vi "combined arm safety.vi"(7 "Input":dbl) -> (8 "Safe Output":dbl, 13 "Safety Data":T1)   [LabVIEW 2013]
uses:
  typedefs/dashboard safety status data.ctl
  typedefs/fg_typedef.ctl
  typedefs/DevRef Type.ctl
  typedefs/subStates.ctl
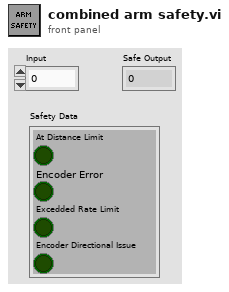
[diagram p1: front panel]
types:
  T1 = typedef "dashboard safety status data.ctl" = cluster{"At Distance Limit":bool, "Encoder Error":bool, "Excedded Rate Limit":bool, "Encoder Directional Issue":bool}
  T2 = typedef "subStates.ctl" = enum16{"null", "wait", "driver control", "auto", "manual override", "hold position", "rotate", "pickup", "pass", "load", "goto shoot", "shoot high goal", "shoot low goal", "cancel arm", "cancel shooter", "end", "test"}
  T3 = typedef "DevRef Type.ctl" = enum16{"Shooter Solenoid", "Latch Solenoid", "Right Up Sensor", "Right Down Sensor", "Hold Sensor", "2 Ball Switch", "Arm Encoder"}
  T4 = typedef "fg_typedef.ctl" = enum16{"Get", "Set"}
  T5 = typedef "WPI_EncoderDevRef.ctl" = cluster{"DevStatus":errorcluster, "EncoderIndex":T6, "CounterIndex":T7, "DistancePerCount":dbl, "Decoding Type":T8}
  T6 = typedef "FPGA_EncoderIdx.ctl" = enum8{"Enc 0", "Enc 1", "Enc 2", "Enc 3", "Invalid"}
  T7 = typedef "FPGA_CounterCtrSystemIndex.ctl" = enum8{"Ctr 0", "Ctr 1", "Ctr 2", "Ctr 3", "Ctr 4", "Ctr 5", "Ctr 6", "Ctr 7", "Invalid"}
  T8 = typedef "WPI_EncoderType.ctl" = enum16{"1x", "2x", "4x"}
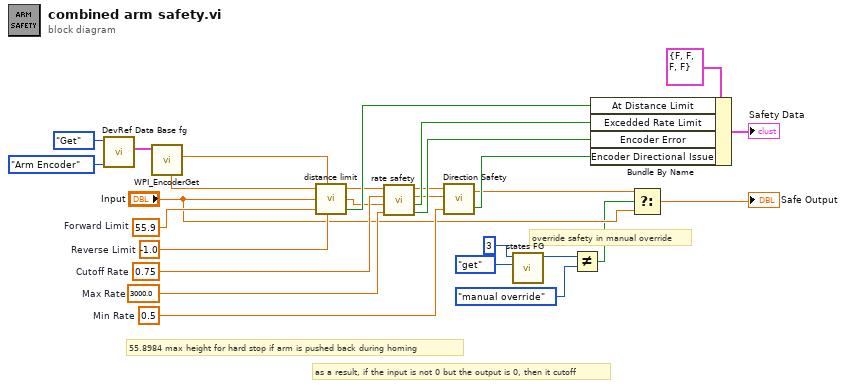
[diagram p0: block diagram]
diagram:
  w21 = 3000.0  # Max Rate
  w20 = 0.5  # Min Rate
  w22 = 0.75  # Cutoff Rate
  w23 = -1.0  # Reverse Limit
  w24 = 55.9  # Forward Limit
  # "override safety in manual override"
  # "55.8984 max height for hard stop if arm is pushed back during homing"
  # "as a result, if the input is not 0 but the output is 0, then it cutoff"
  n1 = call "DevRef Data Base fg.vi"("DevRef to Get"=DevRef_Type."Arm Encoder", "Menu"=fg_typedef."Get") -> ("Selected Encoder"=w27:T5)  [unwired: 2 in, 5 out]
  n2 = call <vilib>:"WPI_EncoderGet.vi"("EncoderDevRef"=w27) -> ("Distance"=w25:dbl, "Rate"=w26:dbl)  [unwired: 5 in, 4 out]
  n3 = call "distance limit.vi"("Encoder Rate"=w26, "Encoder Distance"=w25, "Desired Rate"="Input", "Forward Limit"=w24, "Reverse Limit"=w23) -> ("Encoder Rate Out"=w10:dbl, "Output Rate"=w7:dbl, "At Distance Limit"=w14:bool)
  n4 = call "rate safety.vi"("Max Rate"=w21, "Desired Rate"=w7, "Cutoff Rate"=w22, "Encoder Rate"=w10) -> ("Encoder Error"=w12:bool, "Excedded Rate Limit"=w13:bool, "Output Rate"=w8:dbl, "Encoder Rate Out"=w9:dbl)
  n5 = call "Direction Safety.vi"("Min Rate"=w20, "Desired Rate"=w8, "Encoder Rate"=w9) -> ("Encoder Directional Issue"=w11:bool, "Super Safe Rate"=w3:dbl)
  n6 = call "states FG.vi"("menu (get)"=enum16{"set", "get"}."get", "Loop ID"=3) -> ("subState out"=w6:T2)  [unwired: 6 in, 3 out]
  n7 = Not Equal?(x=w6, y=subStates."manual override") -> (x != y?=w1:bool)
  n8 = Bundle By Name(cluster=T1 {"At Distance Limit"=FALSE, "Encoder Error"=FALSE, "Excedded Rate Limit"=FALSE, "Encoder Directional Issue"=FALSE} ("Input"), "At Distance Limit"=w14, "Excedded Rate Limit"=w13, "Encoder Error"=w12, "Encoder Directional Issue"=w11) -> (→"Safety Data":T1)
  n9 = Select(t=w3, s=w1, f="Input") -> (s? t:f=→"Safe Output":dbl)
